vi "Set Scalar Configuration.vi"(8 "error in (no error)":errorcluster, 9 "index":i32, 10 "thread configuration":T1={"processor"=-2, "priority offset"=0}, 11 "Core Threads Configuration in":refnum<class "Core Threads Configuration.lvclass">) -> (0 "error out":errorcluster, 3 "Core Threads Configuration out":refnum<class "Core Threads Configuration.lvclass">)   [LabVIEW 2017, in "DSF Core.lvlib" / "Core Threads Configuration.lvclass"]
uses:
  Core Threads Configuration.lvclass
  Configuration.ctl
  Core Threads Configuration.lvclass/Core Threads Configuration.ctl
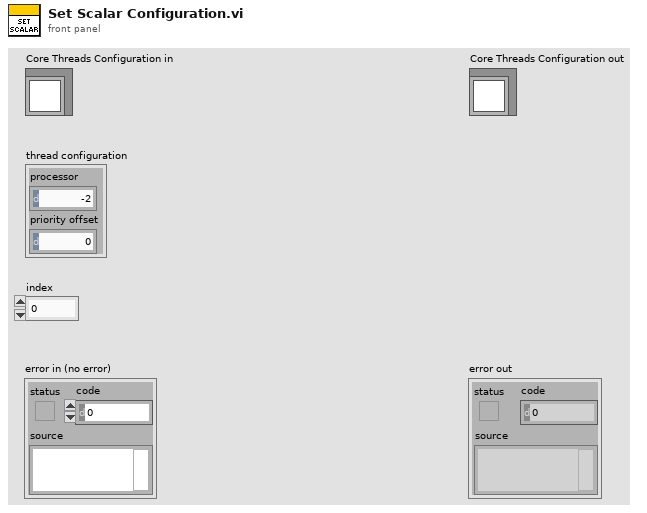
[diagram p1: front panel]
types:
  T1 = typedef "DSF Core.lvlib/Core Threads Configuration.lvclass/Configuration.ctl" = cluster{"processor":i32, "priority offset":i16}
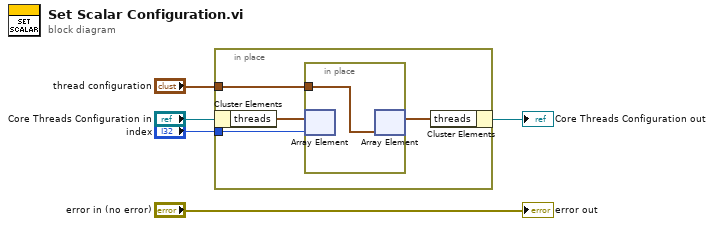
[diagram p0: block diagram]
diagram:
  n1 = in-place {
    in-place-border: "index" -> [w8]
    in-place-border: "thread configuration" -> [w7]
    n2 = in-place-cluster #1("Core Threads Configuration in") -> ("threads"=w9:T1[])
    n3 = in-place {
      in-place-border: w7 -> [w10]
      n4 = in-place-array #2(w9, w8) -> ()  [unwired: 1 out]
      n5 = in-place-array #2(w10) -> (w6:T1[])  [unwired: 1 out]
    }
    n6 = in-place-cluster #1("threads"=w6) -> (→"Core Threads Configuration out":refnum<class "Core Threads Configuration.lvclass">)
  }
  "error out" <- "error in (no error)"
